vi "Write Pulse.vi"(10 "Pulse":refnum<vi>, 11 "Main UI in":refnum<class "Main UI.lvclass">) -> (3 "Main UI out":refnum<class "Main UI.lvclass">)   [LabVIEW 2011, in "Main UI.lvclass"]
uses:
  Main UI.lvclass
  Main UI.lvclass/Main UI.ctl
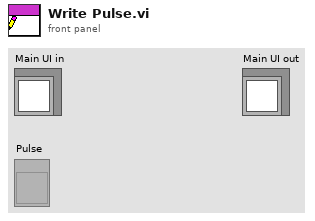
[diagram p1: front panel]
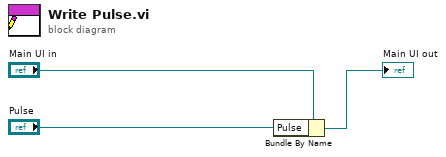
[diagram p0: block diagram]
diagram:
  n1 = Bundle By Name(cluster="Main UI in", "Pulse"="Pulse") -> (→"Main UI out":refnum<class "Main UI.lvclass">)
